vi "古田户外一体站流程平行样自动启动.vi"(9 "参数":T1={"是否启用仪器"=FALSE, "CODMn"={"启动测量模式"={"测量模式"=enum."水样测量"}, "确定按钮"=TRUE}, "启动模块"={"氨氮1"=FALSE, "总磷1"=FALSE, " COD1"=FALSE}, "常规启动"=FALSE, "直接启动"=FALSE}) -> ()   [LabVIEW 2016, in "质控单元.lvlib"]
uses:
  PLC/PLC.lvlib
panel:
  out "COD平行样测完标志":bool
  out "氨氮总磷平行样测完标志":bool
  out "枚举 2":enum16{"初始化", "采配水启动", "等待", "配水", "排水", "结束"}(ring)
  out "枚举":enum16{"初始化", "采配水启动", "等待", "配水", "排水", "结束"}(ring)
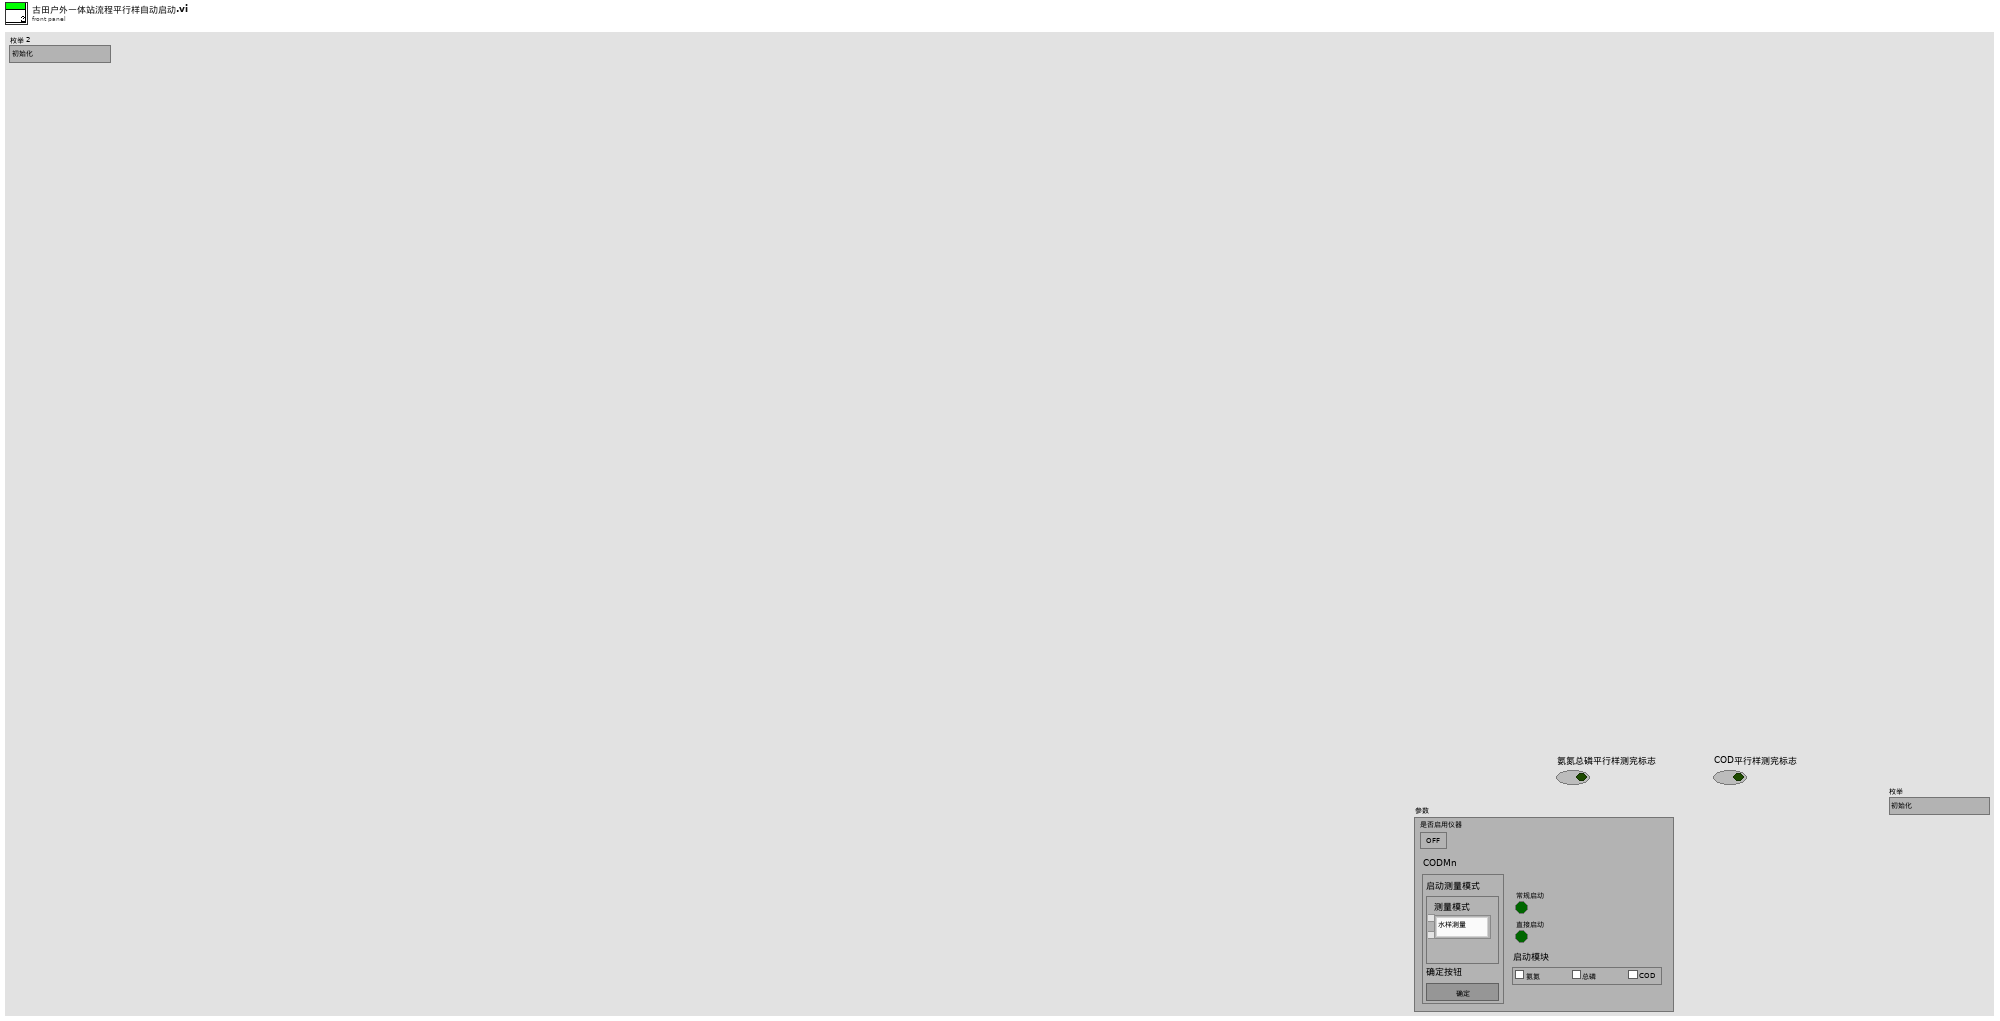
[diagram p1: front panel]
types:
  T1 = cluster{"是否启用仪器":bool, "CODMn":cluster{"启动测量模式":cluster{"测量模式":enum16{"水样测量", "标样核查", "加标回收", "平行样", "校零", "校标"}}, "确定按钮":bool}, "启动模块":cluster{"氨氮1":bool, "总磷1":bool, " COD1":bool}, "常规启动":bool, "直接启动":bool}
  T2 = cluster{"命令":string, cluster{"starting address":u16, "holding register value":u16}}
  T3 = cluster{"R0":i16, "R1":i16, "R2":i16, "R3":i16, "R4":i16, "R5":i16, "R6":i16, "R7":i16, "R8":i16, "R9":i16, "R10":i16, "R11":i16, "R12":i16, "R13":i16, "R14":i16, "R15":i16, "R16":i16, "R17":i16, "R18":i16, "R19":i16, "R20":i16, "R21":i16, "R22":i16, "R23":i16, "R24":i16, "R25":i16}
  T4 = enum32{"Bad", "Idle", "Run top level", "Running"}
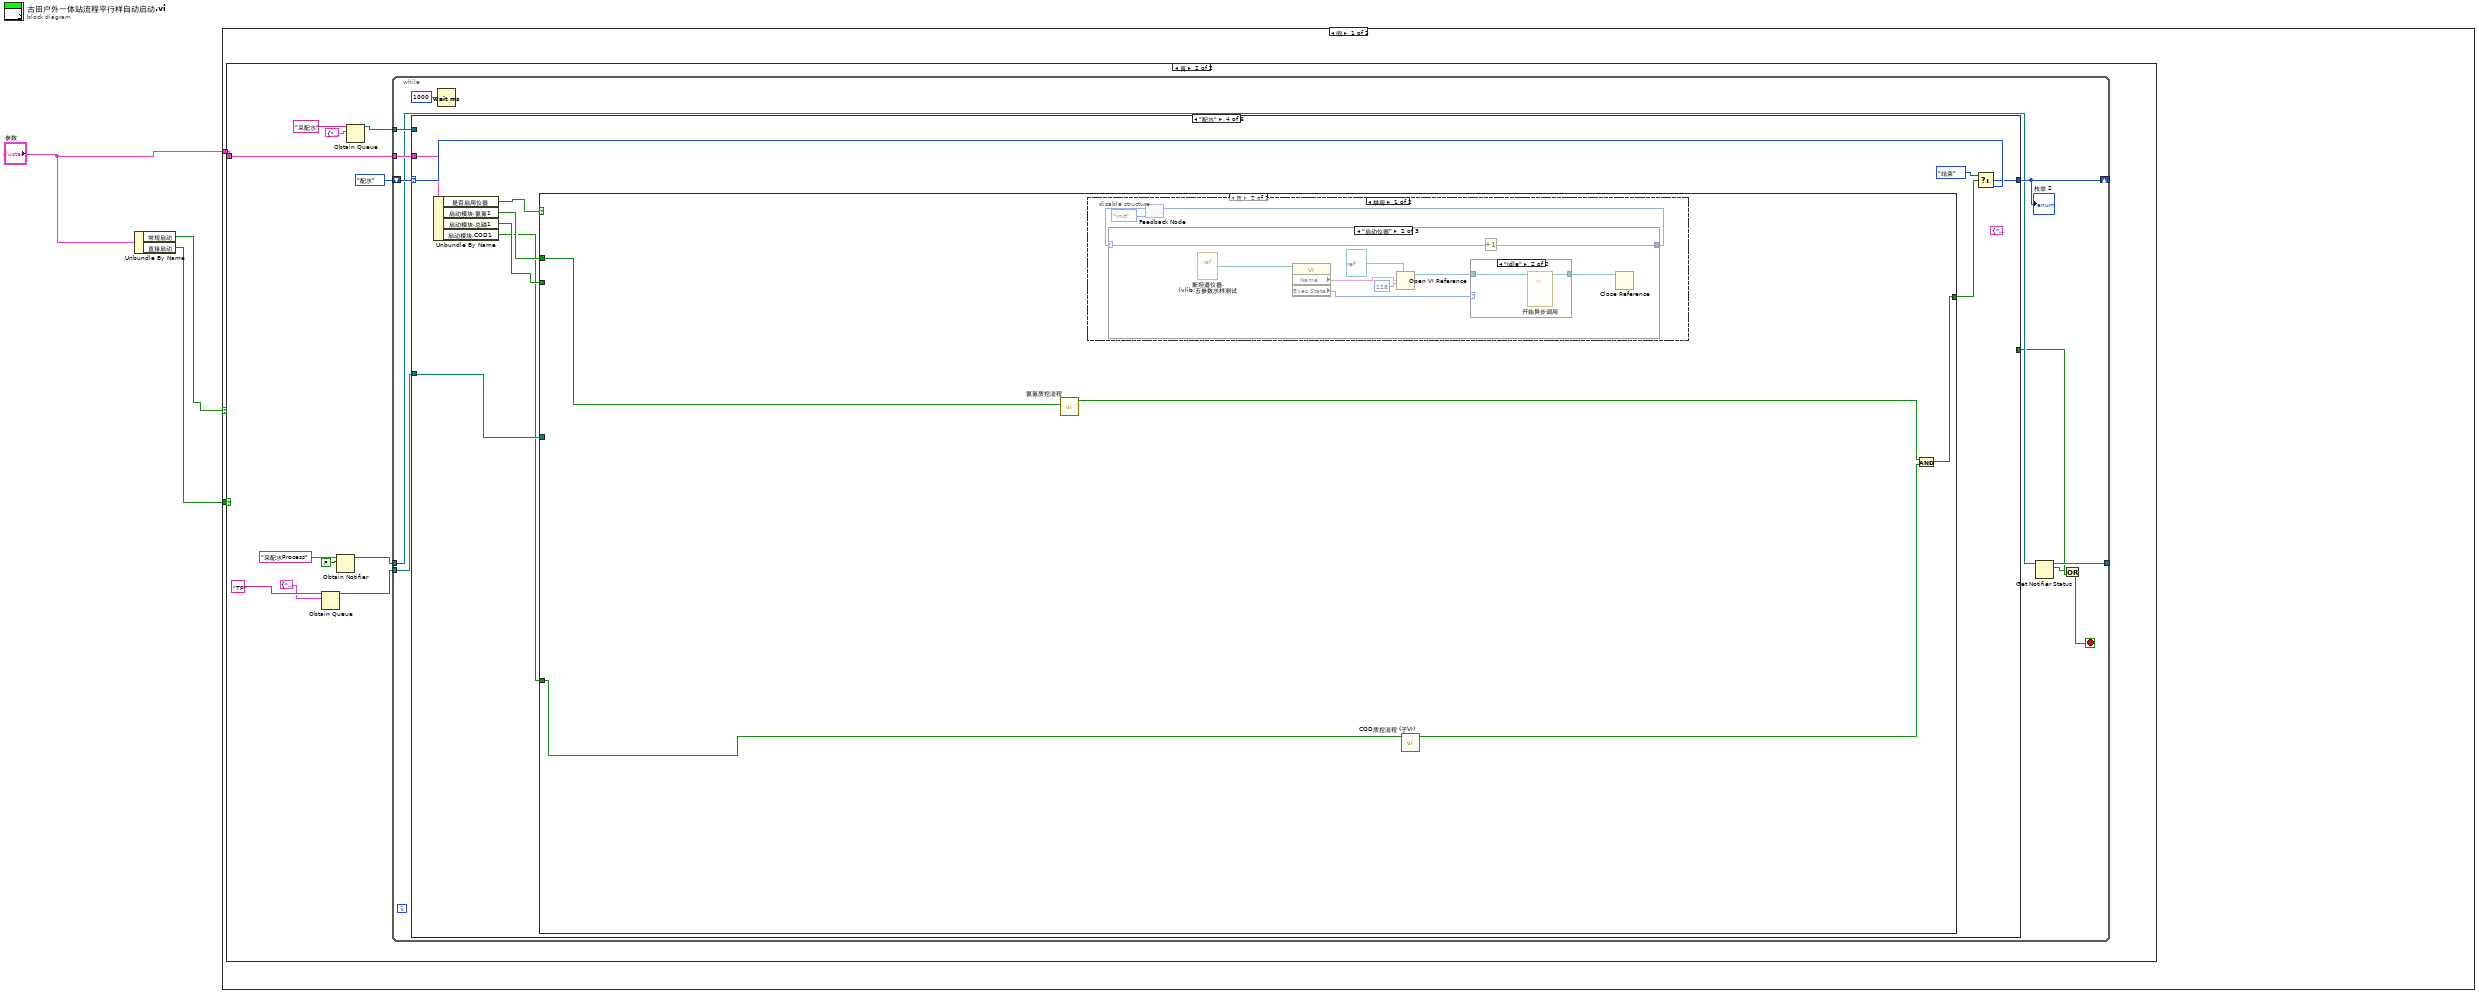
[diagram p0: block diagram]
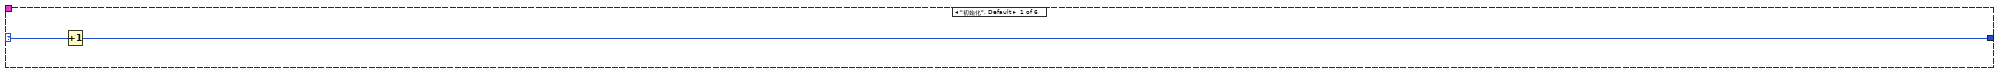
[diagram p3: hidden frame]
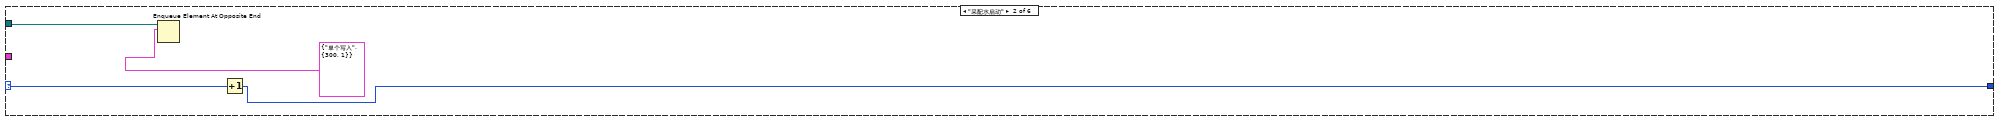
[diagram p4: hidden frame]
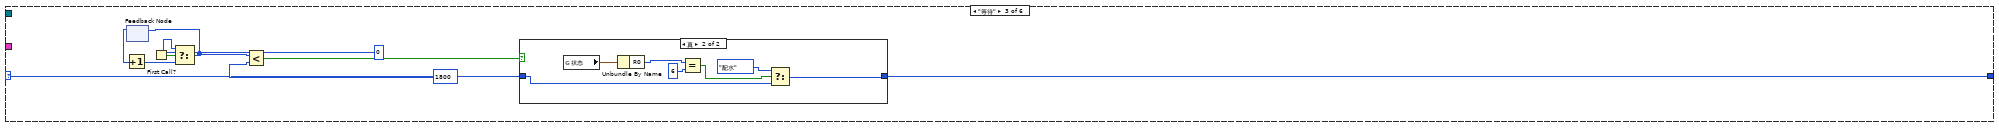
[diagram p5: hidden frame]
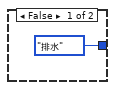
[diagram p6: hidden frame]
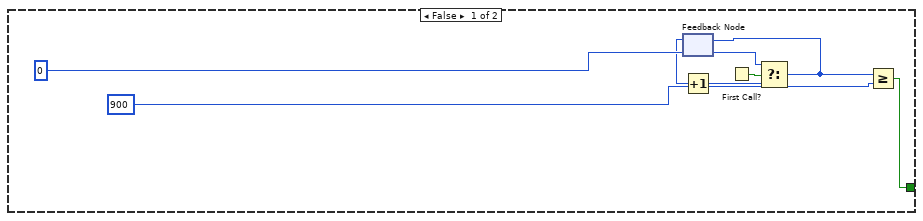
[diagram p7: hidden frame]
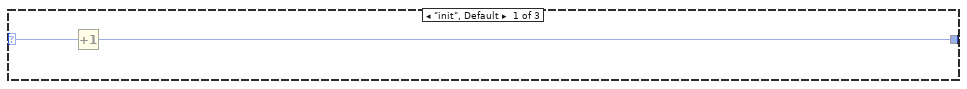
[diagram p8: hidden frame]
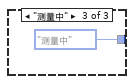
[diagram p10: hidden frame]
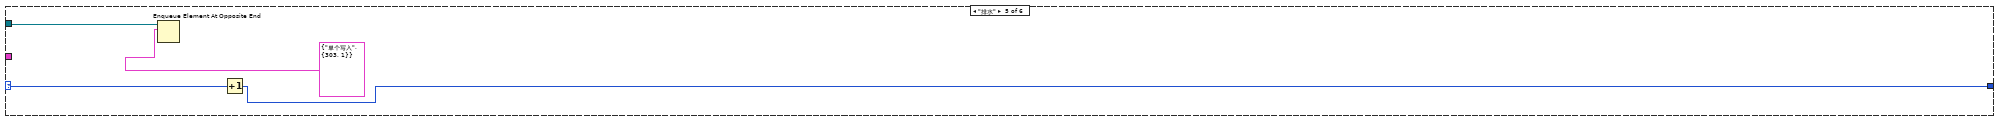
[diagram p12: hidden frame]
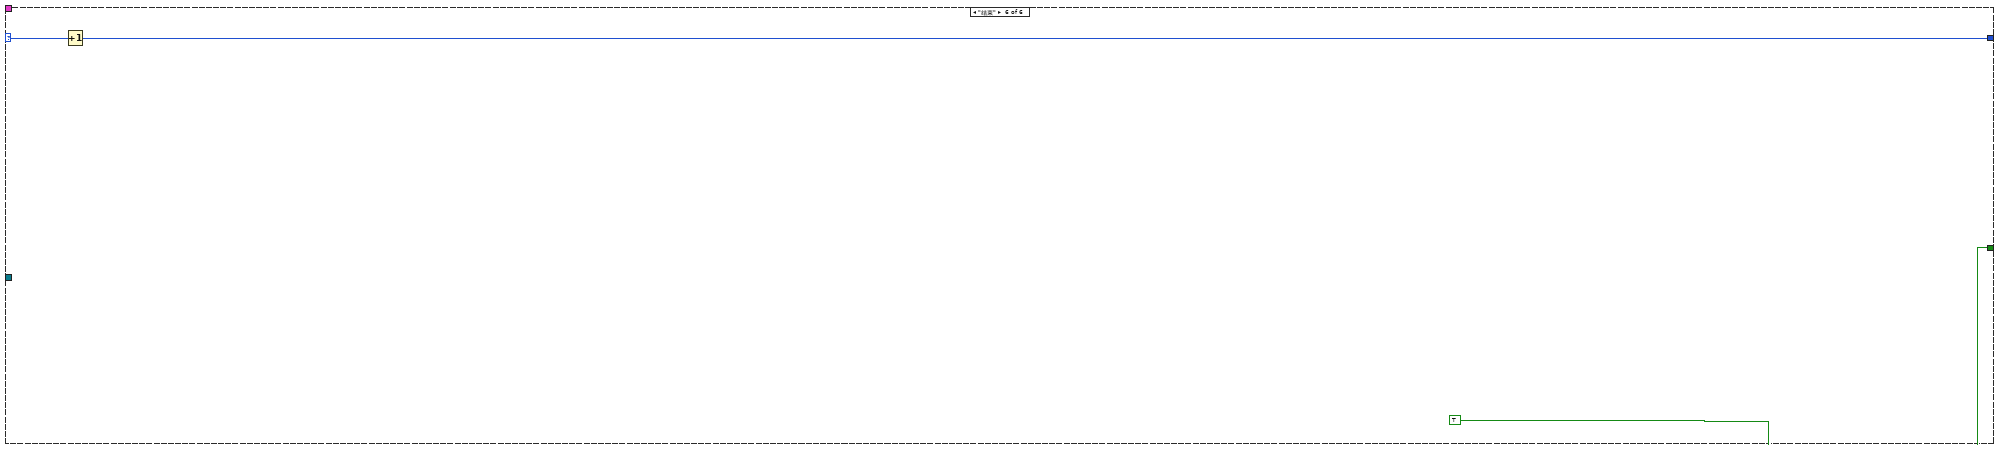
[diagram p13: hidden frame]
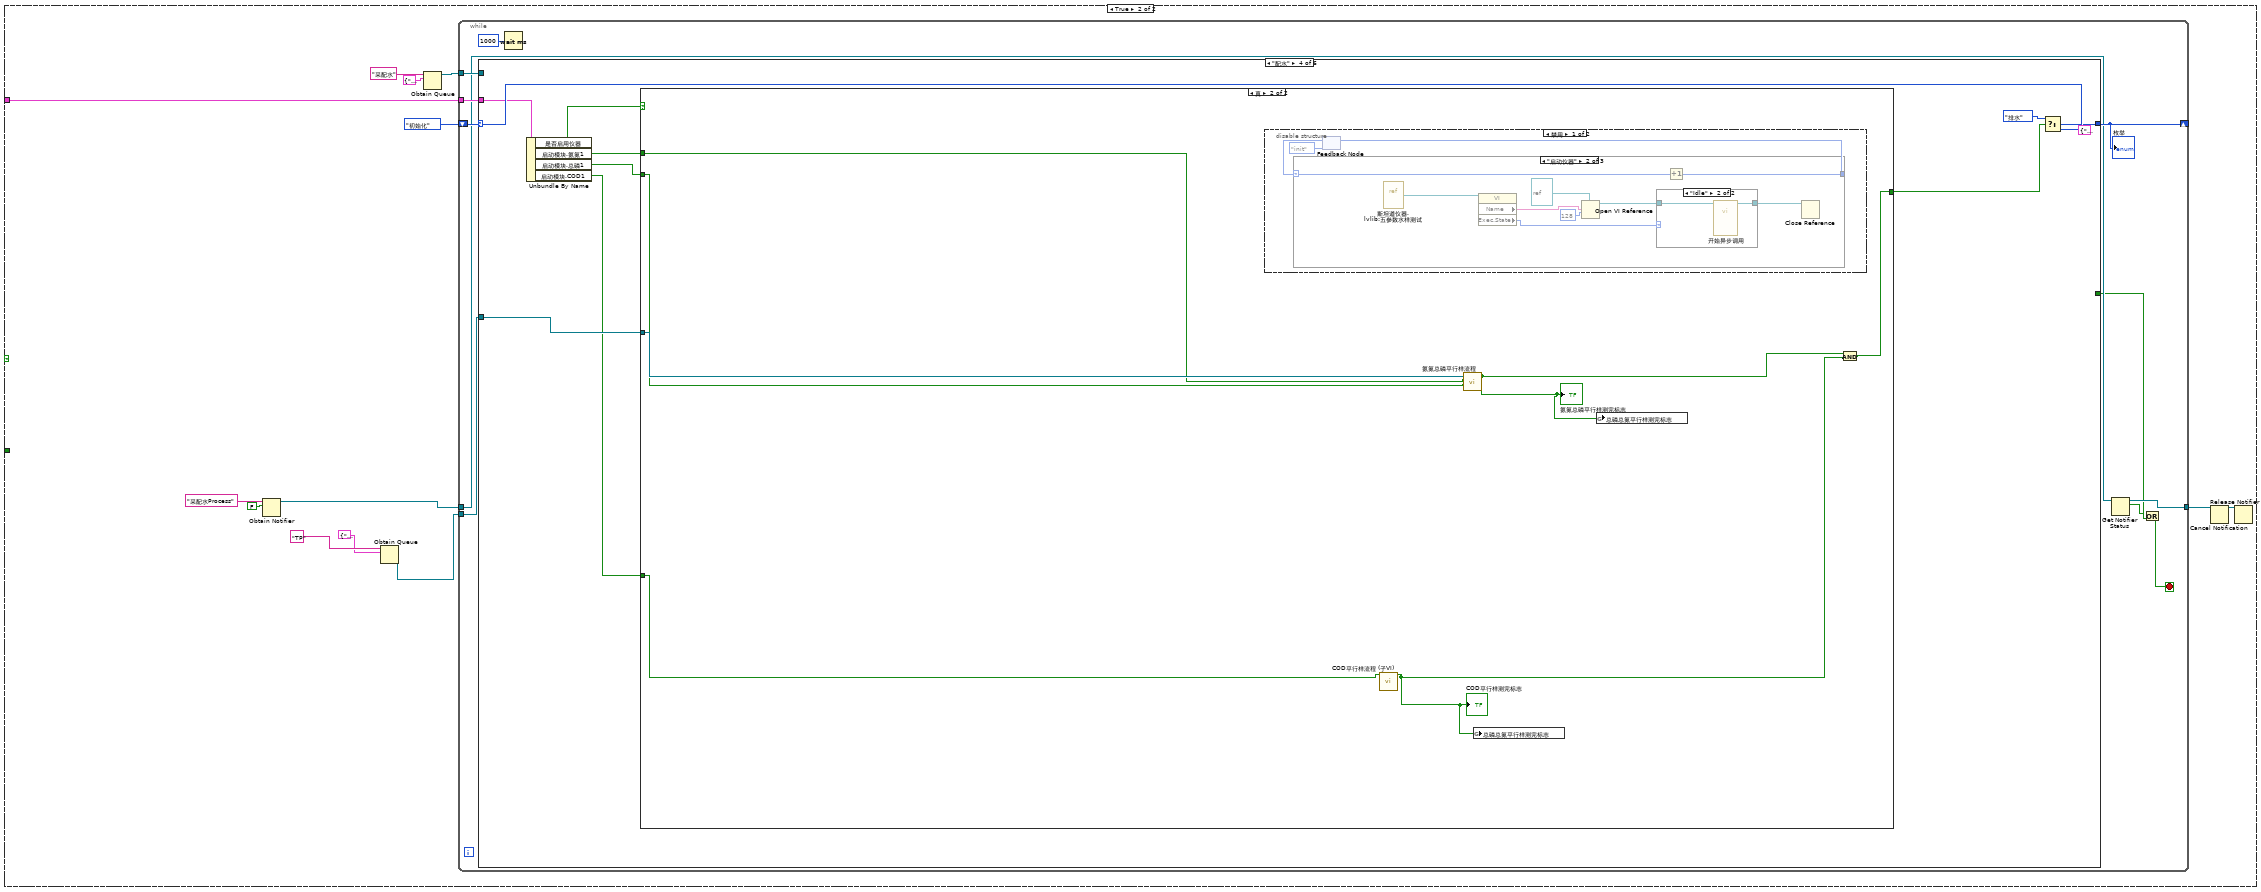
[diagram p14: hidden frame]
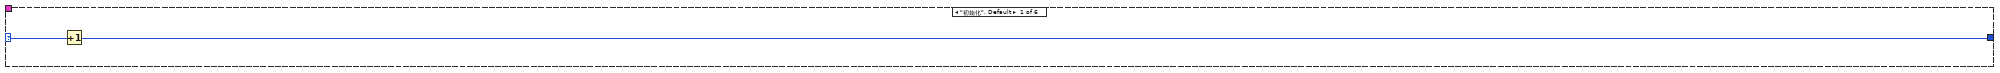
[diagram p15: hidden frame]
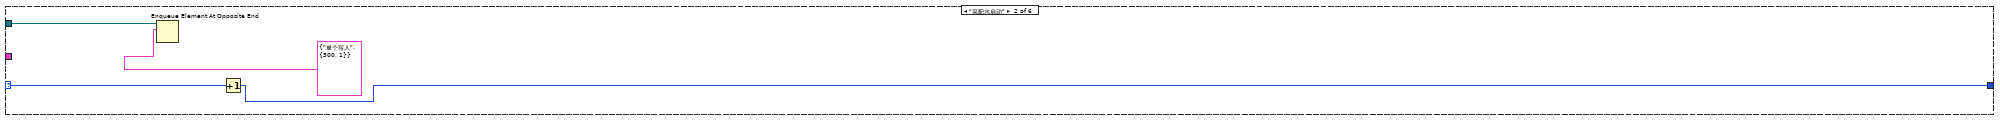
[diagram p16: hidden frame]
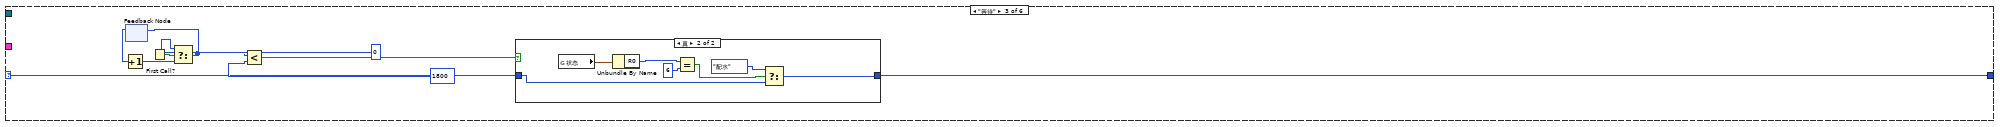
[diagram p17: hidden frame]
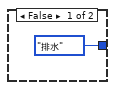
[diagram p18: hidden frame]
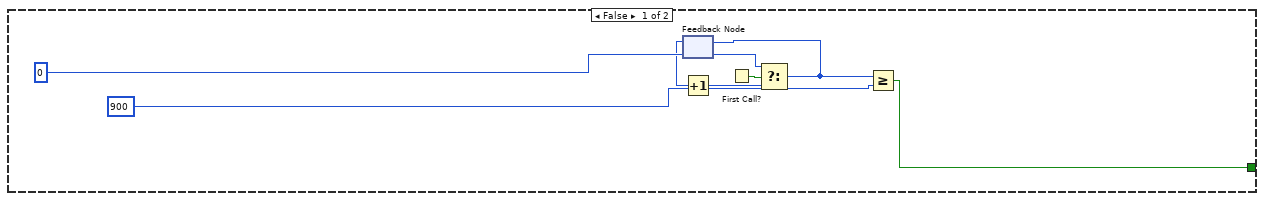
[diagram p19: hidden frame]
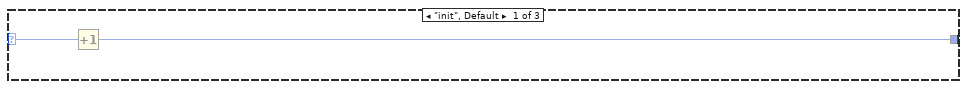
[diagram p20: hidden frame]
diagram:
  n1 = Unbundle By Name("参数") -> ("常规启动"=w2:bool, "直接启动"=w1:bool)
  n2 = case shown="假" w2 {
    tunnel: "参数" -> [w4 w98]
    tunnel: w1 -> [w5 _]
    frame False {
      n3 = case shown="真" w5 {
        tunnel: w4 -> [_ w15]
        frame False {
        }
        frame True {
          n4 = Obtain Queue(name (unnamed)="TP" ("名称（未命名）"), element data type=cluster{"命令":string, "data":variant} {"命令"="", "data"=variant}) -> (queue out=w6:refnum<queue>)  [unwired: 3 in, 2 out]
          n5 = Obtain Notifier(name (unnamed)="采配水Process" ("名称（未命名）"), notification data type=FALSE) -> (notifier out=w9:refnum<notifier>)  [unwired: 2 in, 2 out]
          n6 = Obtain Queue(name (unnamed)="采配水" ("名称（未命名）"), element data type=cluster{"命令":string, "数据":variant} {"命令"="", "数据"=variant}) -> (queue out=w12:refnum<queue>)  [unwired: 3 in, 2 out]
          n7 = while {
            tunnel: w12 -> [w27]
            shift-right: [w25] -> _
            shift-left: enum16{"初始化", "采配水启动", "等待", "配水", "排水", "结束"}."配水" ("枚举") -> [w26]
            tunnel: w6 -> [w23]
            tunnel: w15 -> [w22]
            tunnel: w9 -> [w21]
            tunnel: [w20] -> _
            stop <- w19 stop-if-true
            n8 = case shown="\"配水\"" w26 {
              selector: w26 -> [w29 w31 w40 w59 w92 w97]
              tunnel: w27 -> [_ w32 _ _ w93 _]
              tunnel: [w28 w30 w39 w58 w91 w96] -> w25
              tunnel: [_ _ _ _ _ TRUE] -> w18
              tunnel: w23 -> [_ _ _ w57 _ _]
              tunnel: w22 -> [_ _ _ w54 _ _]
              frame "初始化", Default {
                n9 = Increment(x=w29) -> (x+1=w28:enum16{"初始化", "采配水启动", "等待", "配水", "排水", "结束"})
              }
              frame "采配水启动" {
                n10 = Enqueue Element At Opposite End(queue=w32, element=T2 {"命令"="单个写入", {"starting address"=300, "holding register value"=1}} ("元素")) -> ()  [unwired: 2 in, 3 out]
                n11 = Increment(x=w31) -> (x+1=w30:enum16{"初始化", "采配水启动", "等待", "配水", "排水", "结束"})
              }
              frame "等待" {
                n12 = feedback #1() -> (w36:i32)  [unwired: 1 in]
                n13 = Increment(x=w36) -> (x+1=w35:i32)
                n14 = First Call?() -> (First Call?: T/F=w37:bool)
                n15 = Select(t=0, s=w37, f=w35) -> (s? t:f=w34:i32)
                n16 = feedback-in #1(w34) -> ()
                n17 = Less?(x=w34, y=1800) -> (x < y?=w41:bool)
                n18 = case shown="真" w41 {
                  tunnel: w40 -> [_ w45]
                  tunnel: [enum16{"初始化", "采配水启动", "等待", "配水", "排水", "结束"}."排水" ("枚举") w44] -> w39
                  frame False {
                  }
                  frame True {
                    n19 = global read "采配水全局变量.vi" "状态"() -> (w50:T3)
                    n20 = Unbundle By Name(w50) -> ("R0"=w49:i16)
                    n21 = Equal?(x=w49, y=i16 6) -> (x = y?=w47:bool)
                    n22 = Select(t=enum16{"初始化", "采配水启动", "等待", "配水", "排水", "结束"}."配水" ("枚举"), s=w47, f=w45) -> (s? t:f=w44:enum16{"初始化", "采配水启动", "等待", "配水", "排水", "结束"})
                  }
                }
              }
              frame "配水" {
                (unwired) cluster{"命令":string, "data":variant} {"命令"="启动", "data"=variant(cluster{"站号":u16, "控制命令输出":u16[]} {"站号"=1, "控制命令输出"=[256, 0]})} ("元素")
                n23 = Unbundle By Name(w54) -> ("是否启用仪器"=w56:bool, "启动模块.氨氮1"=w52:bool, "启动模块.总磷1"=w53:bool, "启动模块.COD1"=w51:bool)
                n24 = case shown="真" w56 {
                  tunnel: w57 -> [_ _]
                  tunnel: [w61 w72] -> w55
                  tunnel: w53 -> [_ _]
                  tunnel: w52 -> [_ w70]
                  tunnel: w51 -> [_ w69]
                  frame False {
                    n25 = feedback #2() -> (w65:i32)  [unwired: 1 in]
                    n26 = Increment(x=w65) -> (x+1=w64:i32)
                    n27 = First Call?() -> (First Call?: T/F=w66:bool)
                    n28 = Select(t=0, s=w66, f=w64) -> (s? t:f=w62:i32)
                    n29 = feedback-in #2(w62) -> ()
                    n30 = Greater Or Equal?(x=w62, y=900) -> (x >= y?=w61:bool)
                  }
                  frame True {
                    n31 = call "氨氮质控流程.vi"("氨氮"=w70) -> ("布尔"=w71:bool)  [unwired: 9 in, 1 out]
                    n32 = disable-structure shown="禁用" {
                      frame Disabled {
                        n33 = feedback #3(enum16{"init", "启动仪器", "测量中"}."init") -> (w74:enum16{"init", "启动仪器", "测量中"})
                        n34 = case shown="\"启动仪器\"" w74 {
                          selector: w74 -> [w77 w86 _]
                          tunnel: [w76 w85 enum16{"init", "启动仪器", "测量中"}."测量中"] -> w75
                          frame "init", Default {
                            n35 = Increment(x=w77) -> (x+1=w76:enum16{"init", "启动仪器", "测量中"})
                          }
                          frame "启动仪器" {
                            n36 = vi-ref "斯坦道仪器.lvlib:五参数水样测试.vi"() -> (w78:refnum<vi>)
                            n37 = property class="VI"(reference=w78) -> ("Name"=w82:string, "Exec.State"=w80:T4)  [unwired: 1 in, 2 out]
                            n38 = Open VI Reference(type specifier VI Refnum (for type only)=refnum<vi> refnum ("类型说明符VI引用句柄（仅用于类型）"), vi path=w82, options=128 ("选项")) -> (vi reference=w81:refnum<vi>)  [unwired: 3 in, 1 out]
                            n39 = case shown="\"Idle\"" w80 {
                              tunnel: w81 -> [w87 w89]
                              tunnel: [w87 w88] -> w79
                              frame "Bad", Default {
                              }
                              frame "Idle" {
                                n40 = call-by-ref "开始异步调用"(reference=w89) -> (reference out=w88:refnum<vi>)  [unwired: 13 in, 1 out]
                              }
                            }
                            n41 = Increment(x=w86) -> (x+1=w85:enum16{"init", "启动仪器", "测量中"})
                            n42 = Close Reference(reference=w79) -> ()  [unwired: 1 in, 1 out]
                          }
                          frame "测量中" {
                          }
                        }
                        n43 = feedback-in #3(w75) -> ()
                      }
                      frame Enabled {
                      }
                    }
                    n44 = call "COD质控流程 (子VI).vi"("COD"=w69) -> ("布尔"=w68:bool)  [unwired: 9 in, 1 out]
                    n45 = And(x=w71, y=w68) -> (x .and. y?=w72:bool)
                  }
                }
                n46 = Select(t=enum16{"初始化", "采配水启动", "等待", "配水", "排水", "结束"}."结束" ("枚举"), s=w55, f=w59) -> (s? t:f=w58:enum16{"初始化", "采配水启动", "等待", "配水", "排水", "结束"})
              }
              frame "排水" {
                n47 = Enqueue Element At Opposite End(queue=w93, element=T2 {"命令"="单个写入", {"starting address"=303, "holding register value"=1}} ("元素")) -> ()  [unwired: 2 in, 3 out]
                n48 = Increment(x=w92) -> (x+1=w91:enum16{"初始化", "采配水启动", "等待", "配水", "排水", "结束"})
              }
              frame "结束" {
                n49 = Increment(x=w97) -> (x+1=w96:enum16{"初始化", "采配水启动", "等待", "配水", "排水", "结束"})
              }
            }
            "枚举 2" <- w25
            n50 = Wait (ms)(milliseconds to wait=u32 1000 ("等待时间（毫秒）")) -> ()  [unwired: 1 out]
            n51 = Get Notifier Status(notifier=w21) -> (notifier out=w20:refnum<notifier>, current notification=w17:bool)  [unwired: 1 in, 3 out]
            n52 = Or(x=w17, y=w18) -> (x .or. y?=w19:bool)
          }
        }
      }
    }
    frame True {
      n53 = Obtain Notifier(name (unnamed)="采配水Process" ("名称（未命名）"), notification data type=FALSE) -> (notifier out=w101:refnum<notifier>)  [unwired: 2 in, 2 out]
      n54 = Obtain Queue(name (unnamed)="TP" ("名称（未命名）"), element data type=cluster{"命令":string, "data":variant} {"命令"="", "data"=variant}) -> (queue out=w104:refnum<queue>)  [unwired: 3 in, 2 out]
      n55 = Obtain Queue(name (unnamed)="采配水" ("名称（未命名）"), element data type=cluster{"命令":string, "数据":variant} {"命令"="", "数据"=variant}) -> (queue out=w108:refnum<queue>)  [unwired: 3 in, 2 out]
      n56 = while {
        tunnel: w108 -> [w121]
        shift-right: [w119] -> _
        shift-left: enum16{"初始化", "采配水启动", "等待", "配水", "排水", "结束"}."初始化" ("枚举") -> [w120]
        tunnel: w104 -> [w117]
        tunnel: w98 -> [w116]
        tunnel: w101 -> [w115]
        tunnel: [w114] -> w100
        stop <- w113 stop-if-true
        n57 = case shown="\"配水\"" w120 {
          selector: w120 -> [w123 w125 w134 w153 w188 w193]
          tunnel: w121 -> [_ w126 _ _ w189 _]
          tunnel: [w122 w124 w133 w152 w187 w192] -> w119
          tunnel: [_ _ _ _ _ TRUE] -> w112
          tunnel: w117 -> [_ _ _ w151 _ _]
          tunnel: w116 -> [_ _ _ w148 _ _]
          frame "初始化", Default {
            n58 = Increment(x=w123) -> (x+1=w122:enum16{"初始化", "采配水启动", "等待", "配水", "排水", "结束"})
          }
          frame "采配水启动" {
            n59 = Enqueue Element At Opposite End(queue=w126, element=T2 {"命令"="单个写入", {"starting address"=300, "holding register value"=1}} ("元素")) -> ()  [unwired: 2 in, 3 out]
            n60 = Increment(x=w125) -> (x+1=w124:enum16{"初始化", "采配水启动", "等待", "配水", "排水", "结束"})
          }
          frame "等待" {
            n61 = feedback #4() -> (w130:i32)  [unwired: 1 in]
            n62 = Increment(x=w130) -> (x+1=w129:i32)
            n63 = First Call?() -> (First Call?: T/F=w131:bool)
            n64 = Select(t=0, s=w131, f=w129) -> (s? t:f=w128:i32)
            n65 = feedback-in #4(w128) -> ()
            n66 = Less?(x=w128, y=1800) -> (x < y?=w135:bool)
            n67 = case shown="真" w135 {
              tunnel: w134 -> [_ w139]
              tunnel: [enum16{"初始化", "采配水启动", "等待", "配水", "排水", "结束"}."排水" ("枚举") w138] -> w133
              frame False {
              }
              frame True {
                n68 = global read "采配水全局变量.vi" "状态"() -> (w144:T3)
                n69 = Unbundle By Name(w144) -> ("R0"=w143:i16)
                n70 = Equal?(x=w143, y=i16 6) -> (x = y?=w141:bool)
                n71 = Select(t=enum16{"初始化", "采配水启动", "等待", "配水", "排水", "结束"}."配水" ("枚举"), s=w141, f=w139) -> (s? t:f=w138:enum16{"初始化", "采配水启动", "等待", "配水", "排水", "结束"})
              }
            }
          }
          frame "配水" {
            (unwired) cluster{"命令":string, "data":variant} {"命令"="启动", "data"=variant(cluster{"站号":u16, "控制命令输出":u16[]} {"站号"=1, "控制命令输出"=[256, 0]})} ("元素")
            n72 = Unbundle By Name(w148) -> ("是否启用仪器"=w150:bool, "启动模块.氨氮1"=w146:bool, "启动模块.总磷1"=w147:bool, "启动模块.COD1"=w145:bool)
            n73 = case shown="真" w150 {
              tunnel: w151 -> [_ w168]
              tunnel: [w155 w165] -> w149
              tunnel: w147 -> [_ w166]
              tunnel: w146 -> [_ w167]
              tunnel: w145 -> [_ w164]
              frame False {
                n74 = feedback #5() -> (w159:i32)  [unwired: 1 in]
                n75 = Increment(x=w159) -> (x+1=w158:i32)
                n76 = First Call?() -> (First Call?: T/F=w160:bool)
                n77 = Select(t=0, s=w160, f=w158) -> (s? t:f=w156:i32)
                n78 = feedback-in #5(w156) -> ()
                n79 = Greater Or Equal?(x=w156, y=900) -> (x >= y?=w155:bool)
              }
              frame True {
                n80 = disable-structure shown="禁用" {
                  frame Disabled {
                    n81 = feedback #6(enum16{"init", "启动仪器", "测量中"}."init") -> (w170:enum16{"init", "启动仪器", "测量中"})
                    n82 = case shown="\"启动仪器\"" w170 {
                      selector: w170 -> [w173 w182 _]
                      tunnel: [w172 w181 enum16{"init", "启动仪器", "测量中"}."测量中"] -> w171
                      frame "init", Default {
                        n83 = Increment(x=w173) -> (x+1=w172:enum16{"init", "启动仪器", "测量中"})
                      }
                      frame "启动仪器" {
                        n84 = vi-ref "斯坦道仪器.lvlib:五参数水样测试.vi"() -> (w174:refnum<vi>)
                        n85 = property class="VI"(reference=w174) -> ("Name"=w178:string, "Exec.State"=w176:T4)  [unwired: 1 in, 2 out]
                        n86 = Open VI Reference(type specifier VI Refnum (for type only)=refnum<vi> refnum ("类型说明符VI引用句柄（仅用于类型）"), vi path=w178, options=128 ("选项")) -> (vi reference=w177:refnum<vi>)  [unwired: 3 in, 1 out]
                        n87 = case shown="\"Idle\"" w176 {
                          tunnel: w177 -> [w183 w185]
                          tunnel: [w183 w184] -> w175
                          frame "Bad", Default {
                          }
                          frame "Idle" {
                            n88 = call-by-ref "开始异步调用"(reference=w185) -> (reference out=w184:refnum<vi>)  [unwired: 13 in, 1 out]
                          }
                        }
                        n89 = Increment(x=w182) -> (x+1=w181:enum16{"init", "启动仪器", "测量中"})
                        n90 = Close Reference(reference=w175) -> ()  [unwired: 1 in, 1 out]
                      }
                      frame "测量中" {
                      }
                    }
                    n91 = feedback-in #6(w171) -> ()
                  }
                  frame Enabled {
                  }
                }
                n92 = call "COD平行样流程 (子VI).vi"("COD1"=w164) -> ("布尔"=w162:bool)  [unwired: 10 in]
                "COD平行样测完标志" <- w162
                n93 = call "氨氮总磷平行样流程.vi"("总磷1"=w166, "氨氮1"=w167, "队列输入"=w168) -> ("布尔"=w163:bool)  [unwired: 8 in]
                "氨氮总磷平行样测完标志" <- w163
                n94 = global write "质控测完标志全局 1.vi" "总磷总氮平行样测完标志"(w162) -> ()
                n95 = global write "质控测完标志全局 1.vi" "总磷总氮平行样测完标志"(w163) -> ()
                n96 = And(x=w163, y=w162) -> (x .and. y?=w165:bool)
              }
            }
            n97 = Select(t=enum16{"初始化", "采配水启动", "等待", "配水", "排水", "结束"}."排水" ("枚举"), s=w149, f=w153) -> (s? t:f=w152:enum16{"初始化", "采配水启动", "等待", "配水", "排水", "结束"})
          }
          frame "排水" {
            n98 = Enqueue Element At Opposite End(queue=w189, element=T2 {"命令"="单个写入", {"starting address"=303, "holding register value"=1}} ("元素")) -> ()  [unwired: 2 in, 3 out]
            n99 = Increment(x=w188) -> (x+1=w187:enum16{"初始化", "采配水启动", "等待", "配水", "排水", "结束"})
          }
          frame "结束" {
            n100 = Increment(x=w193) -> (x+1=w192:enum16{"初始化", "采配水启动", "等待", "配水", "排水", "结束"})
          }
        }
        "枚举" <- w119
        n101 = Wait (ms)(milliseconds to wait=u32 1000 ("等待时间（毫秒）")) -> ()  [unwired: 1 out]
        n102 = Get Notifier Status(notifier=w115) -> (notifier out=w114:refnum<notifier>, current notification=w111:bool)  [unwired: 1 in, 3 out]
        n103 = Or(x=w111, y=w112) -> (x .or. y?=w113:bool)
      }
      n104 = Cancel Notification(0:w100) -> (8:w99:refnum<notifier>)  [unwired: 1 in, 2 out]
      n105 = Release Notifier(notifier=w99) -> ()  [unwired: 2 in, 3 out]
    }
  }
